vi "Test Sinewave Module.vi"(8 "error in":errorcluster, 11 "TestCase in":refnum<class "Test FGEN.lvclass">) -> (0 "error out":errorcluster, 3 "TestCase out":refnum<class "Test FGEN.lvclass">)   [LabVIEW 2020, in "Test FGEN.lvclass"]
uses:
  Test FGEN.lvclass
  <vilib>/addons/_JKI Toolkits/VI Tester/TestCase.llb/TestCase.lvclass
  Libraries/FGen/FGen.lvlib
  C:/Program Files (x86)/National Instruments/LabVIEW 2020/vi.lib/addons/_JKI Toolkits/VI Tester/TestCase.llb/TestCase.lvclass
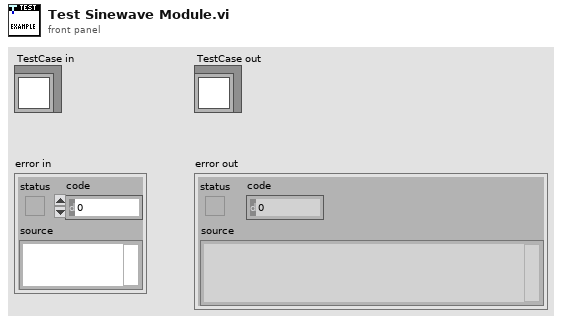
[diagram p1: front panel]
types:
  T1 = typedef "FGen.lvlib/Generate Signal (Reply Payload)--cluster.ctl" = cluster{"signal out":waveform(dbl), "Generate Signal_error":errorcluster}
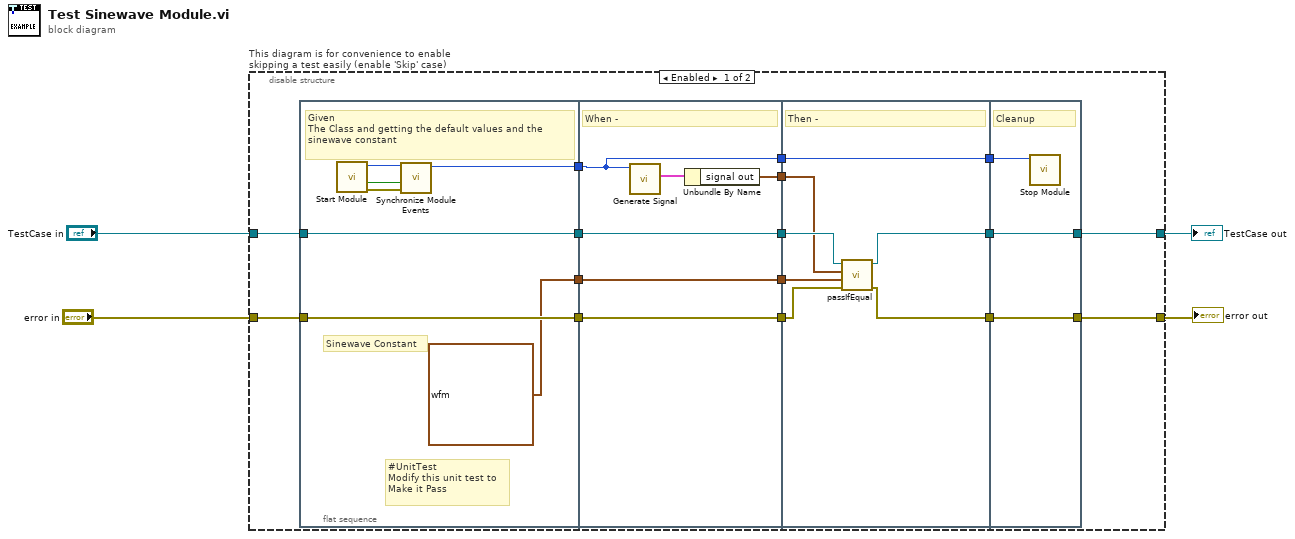
[diagram p0: block diagram]
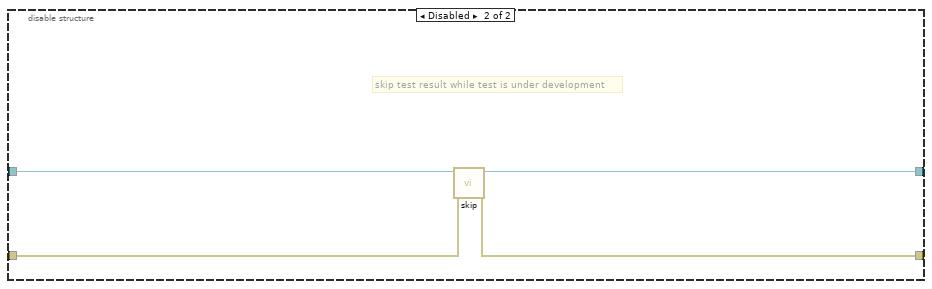
[diagram p2: hidden frame]
diagram:
  n1 = disable-structure "This diagram is for convenience to enable skipping a test easily (enable 'Skip' case)" shown="Enabled" {
    disable-tunnel: "TestCase in" -> [w12 w45]
    disable-tunnel: [w11 w44] -> w1
    disable-tunnel: [w19 w47] -> w3
    disable-tunnel: "error in" -> [w18 w46]
    frame Enabled {
      n2 = flat-sequence {
        tunnel: w12 -> [w25]
        tunnel: [w25] -> w15
        tunnel: w18 -> [w27]
        tunnel: [w27] -> w16
        tunnel: [w23] -> w10
        tunnel: [waveform(dbl) {"t0"=timestamp(0 s since 1904-01-01), "dt"=1.0, "Y"=[]} ("signal out")] -> w5
        tunnel: [w32] -> w14
        tunnel: w15 -> [w32]
        tunnel: [w33] -> w17
        tunnel: w16 -> [w33]
        tunnel: w10 -> [w29]
        tunnel: [w30] -> w9
        tunnel: [w29] -> w8
        tunnel: [w28] -> w6
        tunnel: w5 -> [w28]
        tunnel: [w37] -> w13
        tunnel: [w40] -> w20
        tunnel: w14 -> [w38]
        tunnel: w17 -> [w39]
        tunnel: w9 -> [w36]
        tunnel: w8 -> [w35]
        tunnel: [w35] -> w7
        tunnel: w6 -> [w34]
        tunnel: [w43] -> w19
        tunnel: [w42] -> w11
        tunnel: w13 -> [w42]
        tunnel: w20 -> [w43]
        tunnel: w7 -> [w41]
        frame #0 {
          # "Sinewave Constant"
          # "#UnitTest\nModify this unit test to\nMake it Pass"
          # "Given\nThe Class and getting the default values and the sinewave constant"
          n3 = call "Start Module.vi"() -> ("error out"=w26:errorcluster, "Wait for Event Sync?"=w22:bool, "Module ID"=w24:i32)  [unwired: 8 in, 1 out]
          n4 = call "Synchronize Module Events.vi"("error in"=w26, "Wait for Event Sync?"=w22, "Module ID in"=w24) -> ("Module ID out"=w23:i32)  [unwired: 7 in, 1 out]
        }
        frame #1 {
          # "When -"
          n5 = call "Generate Signal.vi"("Module ID"=w29) -> ("Reply Payload"=w31:T1)  [unwired: 8 in, 2 out]
          n6 = Unbundle By Name(w31) -> ("signal out"=w30:waveform(dbl))
        }
        frame #2 {
          # "Then -"
          n7 = call-dynamic "passIfEqual.vi"("error in (no error)"=w39, "y"=w34, "x"=w36, "TestCase in"=w38) -> ("error out"=w40:errorcluster, "TestCase out"=w37:refnum<class "Test FGEN.lvclass">)  [unwired: 6 in]
        }
        frame #3 {
          # "Cleanup"
          n8 = call "Stop Module.vi"("Module ID"=w41) -> ()  [unwired: 10 in, 1 out]
        }
      }
    }
    frame Disabled {
      # "skip test result while test is under development"
      n9 = call <vilib>:"skip.vi"("error in (no error)"=w46, "TestCase in"=w45) -> ("error out"=w47:errorcluster, "TestCase out"=w44:refnum<class "Test FGEN.lvclass">)  [unwired: 8 in]
    }
  }
  "error out" <- w3
  "TestCase out" <- w1
